vi "Displace-relative.vi"(8 "error in (no error)":errorcluster, 9 "Min duration":dbl caption="Min. duration [s]", 10 "Displacement":dbl caption="Displacement [unit]", 11 "Motor-Maxon in":refnum<class "Motor-Maxon.lvclass">) -> (0 "error out":errorcluster, 3 "Motor-Maxon out":refnum<class "Motor-Maxon.lvclass">)   [LabVIEW 2013, in "PowderDeposition.lvlib" / "Motor-Maxon.lvclass"]
uses:
  Motor-Maxon.lvclass
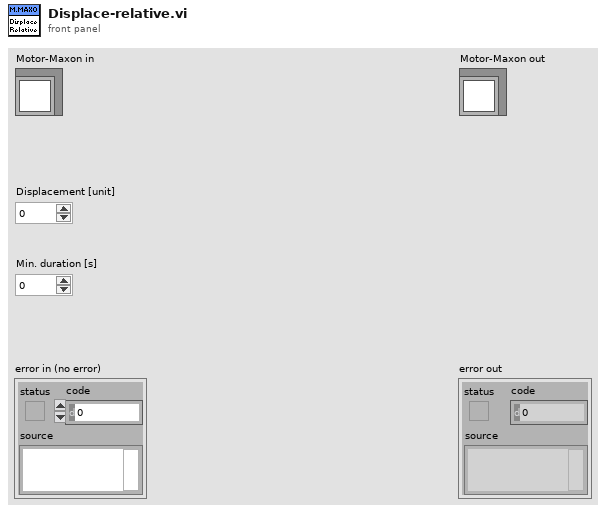
[diagram p1: front panel]
types:
  T1 = cluster{"profileVelocity":u32, "profileAcceleration":u32, "profileDeceleration":u32}
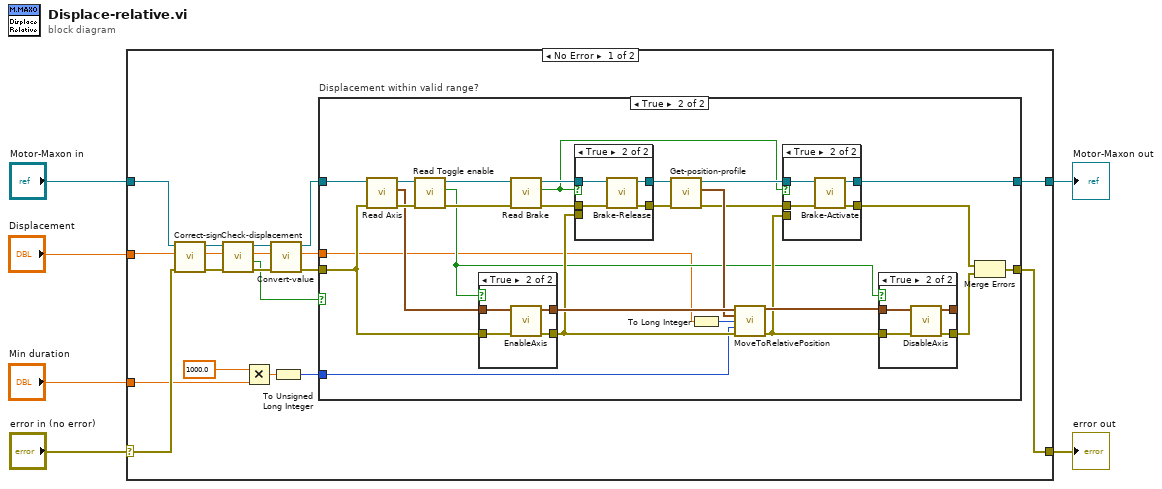
[diagram p0: block diagram]
diagram:
  n1 = case shown="No Error" "error in (no error)" {
    selector: "error in (no error)" -> [w19 w80]
    tunnel: [w11 w80] -> w5
    tunnel: [w25 w79] -> w3
    tunnel: "Motor-Maxon in" -> [w17 w79]
    tunnel: "Displacement" -> [w24 _]
    tunnel: "Min duration" -> [w8 _]
    frame No Error {
      n2 = call-dynamic "Correct-sign.vi"("error in (no error)"=w19, "Value in"=w24, "Motor in"=w17) -> ("error out"=w21:errorcluster, "Value out"=w23:dbl, "Motor out"=w14:refnum<class "Motor-Maxon.lvclass">)  [unwired: 6 in]
      n3 = call-dynamic "Check-displacement.vi"("error in (no error)"=w21, "Displacement in"=w23, "Motor-Serial in"=w14) -> ("error out"=w20:errorcluster, "In range?"=w13:bool, "Displacement out"=w22:dbl, "Motor-Serial out"=w15:refnum<class "Motor-Maxon.lvclass">)  [unwired: 5 in]
      n4 = Multiply(x=1000.0, y=w8) -> (x*y=w9:dbl)
      n5 = call-dynamic "Convert-value.vi"("error in (no error)"=w20, "Value in"=w22, "Motor-Serial in"=w15) -> ("error out"=w18:errorcluster, "Value out"=w12:dbl, "Motor-Serial out"=w16:refnum<class "Motor-Maxon.lvclass">)  [unwired: 6 in]
      n6 = To Unsigned Long Integer(number=w9) -> (unsigned 32bit integer=w7:u32)
      n7 = case "Displacement within valid range?" shown="True" w13 {
        tunnel: [w27 w32] -> w25
        tunnel: w18 -> [w26 w42]
        tunnel: w16 -> [w27 w41]
        tunnel: w12 -> [_ w34]
        tunnel: [w26 w31] -> w11
        tunnel: w7 -> [_ w28]
        frame False {
        }
        frame True {
          n8 = call-dynamic "Read Axis.vi"("error in (no error)"=w42, "Motor-Maxon in"=w41) -> ("error out"=w53:errorcluster, "Axis"=w52:cluster{"keyHandle":u32, "nodeID":u16}, "Motor-Maxon out"=w54:refnum<class "Motor-Maxon.lvclass">)  [unwired: 7 in]
          n9 = call-dynamic "Read Toggle enable.vi"("error in (no error)"=w53, "Motor-Maxon in"=w54) -> ("error out"=w50:errorcluster, "Toggle enable"=w35:bool, "Motor-Maxon out"=w51:refnum<class "Motor-Maxon.lvclass">)  [unwired: 7 in]
          n10 = case shown="True" w35 {
            tunnel: w52 -> [w74 w77]
            tunnel: w42 -> [w73 w78]
            tunnel: [w74 w76] -> w47
            tunnel: [w73 w75] -> w46
            frame False {
            }
            frame True {
              n11 = call <instrlib>:"EnableAxis.vi"("error in (no error)"=w78, "axis in"=w77) -> ("error out"=w75:errorcluster, "axis out"=w76:cluster{"keyHandle":u32, "nodeId":u16})  [unwired: 4 in]
            }
          }
          n12 = call-dynamic "Read Brake.vi"("error in (no error)"=w50, "Motor-Maxon in"=w51) -> ("error out"=w48:errorcluster, "Brake"=w38:bool, "Motor-Maxon out"=w49:refnum<class "Motor-Maxon.lvclass">)  [unwired: 7 in]
          n13 = case shown="True" w38 {
            tunnel: w49 -> [w68 w72]
            tunnel: w48 -> [w67 w71]
            tunnel: [w68 w70] -> w45
            tunnel: [w67 w69] -> w44
            tunnel: w46 -> [_ _]
            frame False {
            }
            frame True {
              n14 = call-dynamic "Brake-Release.vi"("error in (no error)"=w71, "Motor-Maxon in"=w72) -> ("error out"=w69:errorcluster, "Motor-Maxon out"=w70:refnum<class "Motor-Maxon.lvclass">)  [unwired: 8 in]
            }
          }
          n15 = call-dynamic "Get-position-profile.vi"("error in (no error)"=w44, "Motor-Maxon in"=w45) -> ("error out"=w39:errorcluster, "Position profile"=w43:T1, "Motor-Maxon out"=w40:refnum<class "Motor-Maxon.lvclass">)  [unwired: 7 in]
          n16 = To Long Integer(number=w34) -> (32bit integer=w33:i32)
          n17 = call <instrlib>:"MoveToRelativePosition.vi"("axis in"=w47, "position profile"=w43, "relative position"=w33, "timeout"=w28, "error in (no error)"=w46) -> ("axis out"=w37:cluster{"keyHandle":u32, "nodeId":u16}, "error out"=w36:errorcluster)  [unwired: 9 in]
          n18 = case shown="True" w38 {
            tunnel: w40 -> [w56 w58]
            tunnel: w39 -> [w55 w57]
            tunnel: [w56 w59] -> w32
            tunnel: [w55 w60] -> w30
            tunnel: w36 -> [_ _]
            frame False {
            }
            frame True {
              n19 = call-dynamic "Brake-Activate.vi"("error in (no error)"=w57, "Motor-Maxon in"=w58) -> ("error out"=w60:errorcluster, "Motor-Maxon out"=w59:refnum<class "Motor-Maxon.lvclass">)  [unwired: 8 in]
            }
          }
          n20 = case shown="True" w35 {
            tunnel: w37 -> [w62 w63]
            tunnel: w36 -> [w61 w64]
            tunnel: [w62 w66] -> _
            tunnel: [w61 w65] -> w29
            frame False {
            }
            frame True {
              n21 = call <instrlib>:"DisableAxis.vi"("error in (no error)"=w64, "axis in"=w63) -> ("error out"=w65:errorcluster, "axis out"=w66:cluster{"keyHandle":u32, "nodeId":u16})  [unwired: 4 in]
            }
          }
          n22 = Merge Errors(w30, w29) -> (w31:errorcluster)
        }
      }
    }
    frame Error {
    }
  }
  "error out" <- w5
  "Motor-Maxon out" <- w3
